vi "Plot current data.vi"(9 "file path (dialog if empty)":path) -> (1 "XY Graph":cluster{"Y":dbl[], "Y":dbl[]}[](graph))   [LabVIEW 2011]
uses:
  <vilib>/Utility/file.llb/Read From Spreadsheet File (DBL).vi
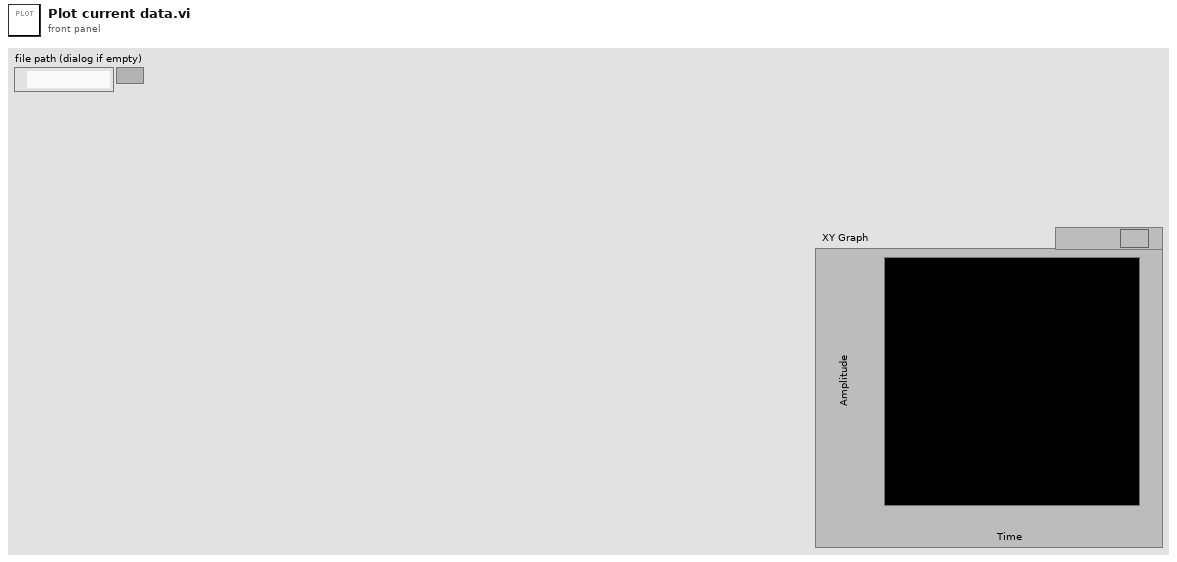
[diagram p1: front panel]
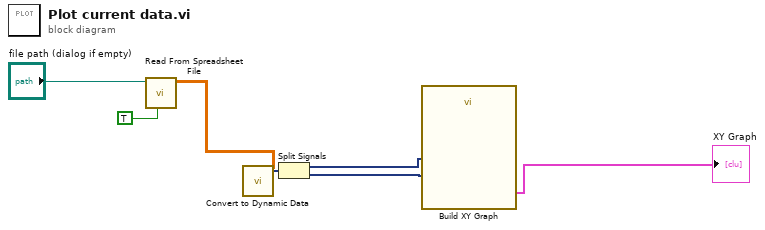
[diagram p0: block diagram]
diagram:
  n1 = call-poly <vilib>:"Read From Spreadsheet File.vi"("transpose (no:F)"=TRUE, "file path (dialog if empty)"="file path (dialog if empty)") -> ("all rows"=w4:dbl[][])  [unwired: 5 in, 4 out]
  n2 = call "Convert to Dynamic Data"("2D Array"=w4) -> ("Dynamic Data Type"=w5:dynamicdata)  [unwired: 3 in]
  n3 = Split Signals(w5) -> (w1:dynamicdata, w6:dynamicdata)  [unwired: 2 in]
  n4 = call "Build XY Graph"("Y Input"=w6, "X Input"=w1) -> ("XY Graph"=→"XY Graph":cluster{"Y":dbl[], "Y":dbl[]}[])  [unwired: 3 in, 6 out]
